vi "Update DMA Values - 321.vi"(8 "error in (no error)":errorcluster, 11 "Register Value":variant) -> (0 "error out":errorcluster, 3 "Updated DMA Values":T1[](array[typedef]) {"Data Type" format="%.0x"})   [LabVIEW 2018, in "FPGA Addon Shared.lvlib"]
uses:
  FPGA Addon Shared.lvlib
  Types/DMA Information.ctl
  Types/FPGA Addon Data Type.ctl
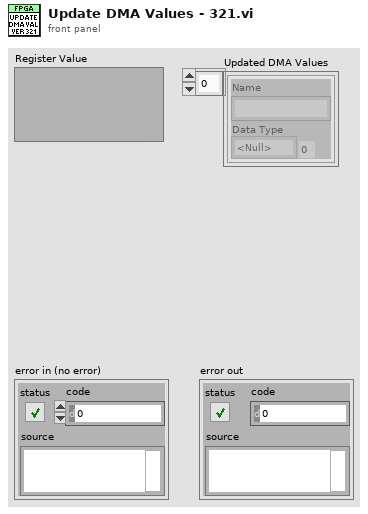
[diagram p1: front panel]
types:
  T1 = typedef "FPGA Addon Shared.lvlib/DMA Information.ctl" = cluster{"Name":string, "Data Type":T2}
  T2 = typedef "FPGA Addon Shared.lvlib/FPGA Addon Data Type.ctl" = enum8{"<Null>", "I8", "I16", "I32", "I64", "U8", "U16", "U32", "U64", "SGL", "Boolean", "Analog PWM In Settings", "Analog PWM In", "Digital PWM In Settings", "Digital PWM In", "Digital PWM Out", "Sine Out", "FXP", "FXP+/-24.5", "FXP+/-16.5", "FXP+/-32.8", "FXP+/-64.32", "FXP+/-16.7", "FXP+/-20.5", "FXP+/-27.5", "FXP+/-32.16", "FXP+16.3", "FXP+18.3", "Digital Static In", "Digital Static Out", "Digital Static In Settings", "Digital WSS Out", "Quad Encoder Settings", "Quad Encoder In", "Group"}
  T3 = cluster{"Name":string, "Data Type":enum8{"<Null>", "I8", "I16", "I32", "I64", "U8", "U16", "U32", "U64", "SGL", "Boolean", "Analog PWM In Settings", "Analog PWM In", "Digital PWM In Settings", "Digital PWM In", "Digital PWM Out", "Sine Out", "FXP+/-24.5", "FXP+/-16.5", "FXP+/-32.8", "FXP+/-64.32", "FXP+/-16.7", "FXP+/-20.5", "FXP+/-27.5", "FXP+/-32.16", "FXP+16.3", "FXP+18.3", "Digital Static In", "Digital Static Out", "Digital Static In Settings", "Digital WSS Out", "Quad Encoder Settings", "Quad Encoder In", "Group"}}[]
  T4 = enum8{"<Null>", "I8", "I16", "I32", "I64", "U8", "U16", "U32", "U64", "SGL", "Boolean", "Analog PWM In Settings", "Analog PWM In", "Digital PWM In Settings", "Digital PWM In", "Digital PWM Out", "Sine Out", "FXP+/-24.5", "FXP+/-16.5", "FXP+/-32.8", "FXP+/-64.32", "FXP+/-16.7", "FXP+/-20.5", "FXP+/-27.5", "FXP+/-32.16", "FXP+16.3", "FXP+18.3", "Digital Static In", "Digital Static Out", "Digital Static In Settings", "Digital WSS Out", "Quad Encoder Settings", "Quad Encoder In", "Group"}
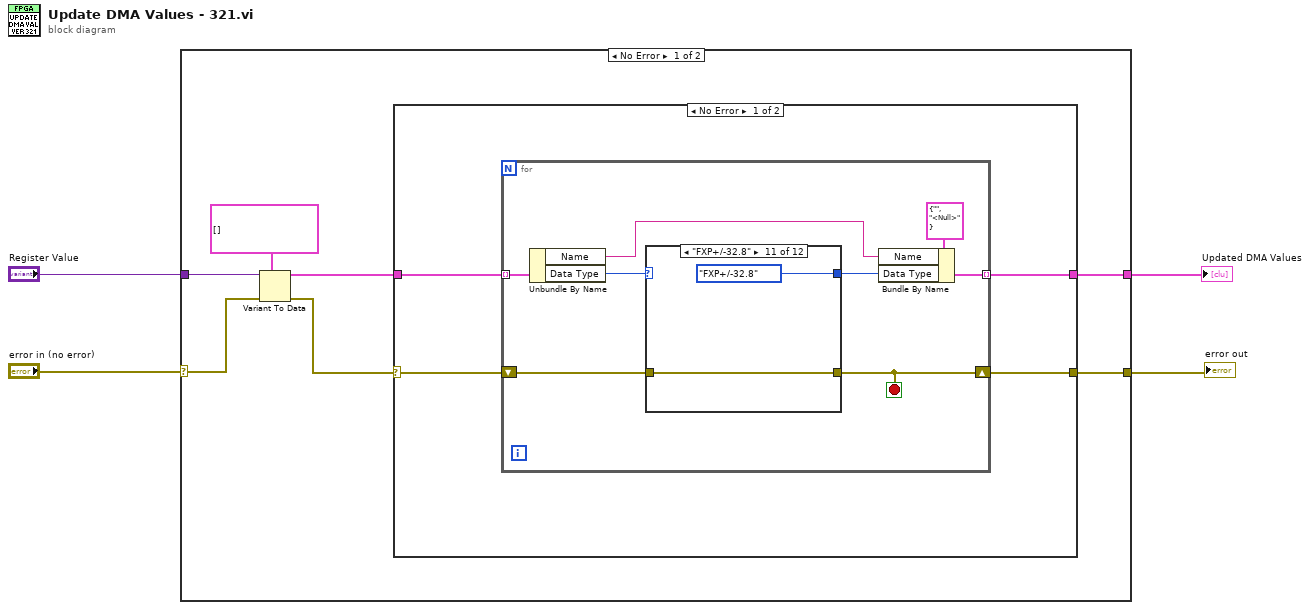
[diagram p0: block diagram]
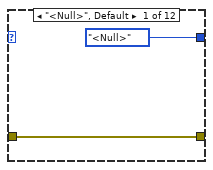
[diagram p2: hidden frame]
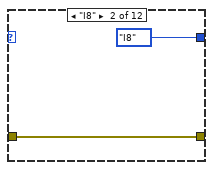
[diagram p3: hidden frame]
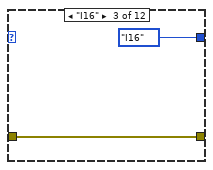
[diagram p4: hidden frame]
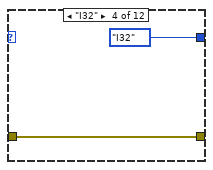
[diagram p5: hidden frame]
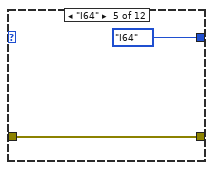
[diagram p6: hidden frame]
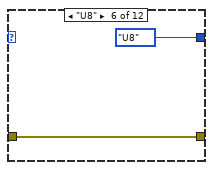
[diagram p7: hidden frame]
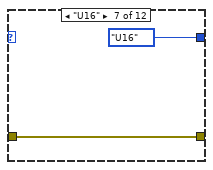
[diagram p8: hidden frame]
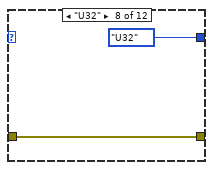
[diagram p9: hidden frame]
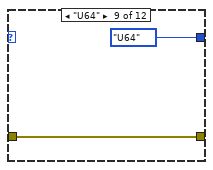
[diagram p10: hidden frame]
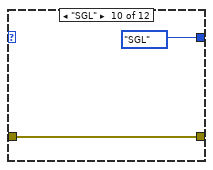
[diagram p11: hidden frame]
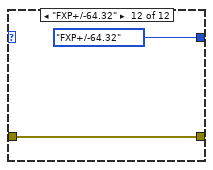
[diagram p12: hidden frame]
diagram:
  n1 = case shown="No Error" "error in (no error)" {
    selector: "error in (no error)" -> [w8 w49]
    tunnel: [w11 _] -> w1
    tunnel: "Register Value" -> [w9 _]
    tunnel: [w6 w49] -> w2
    frame No Error {
      n2 = Variant To Data(error in=w8, type=T3 [] ("Available DMA"), Variant=w9) -> (data=w10:T3, error out=w7:errorcluster)
      n3 = case shown="No Error" w7 {
        selector: w7 -> [w13 w48]
        tunnel: [w15 _] -> w11
        tunnel: w10 -> [w14 _]
        tunnel: [w12 w48] -> w6
        frame No Error {
          n4 = for {
            tunnel: w14 -> [w23] mode=indexing
            tunnel: [w22] -> w15 mode=indexing
            shift-right: [w18] -> w12
            shift-left: w13 -> [w19]
            stop <- w18 stop-if-true
            n5 = Unbundle By Name(w23) -> ("Name"=w17:string, "Data Type"=w21:T4)
            n6 = case shown="\"FXP+/-32.8\"" w21 {
              tunnel: [FPGA_Addon_Data_Type."<Null>" ("Data Type") FPGA_Addon_Data_Type."I8" ("Data Type") FPGA_Addon_Data_Type."I16" ("Data Type") FPGA_Addon_Data_Type."I32" ("Data Type") FPGA_Addon_Data_Type."I64" ("Data Type") FPGA_Addon_Data_Type."U8" ("Data Type") FPGA_Addon_Data_Type."U16" ("Data Type") FPGA_Addon_Data_Type."U32" ("Data Type") FPGA_Addon_Data_Type."U64" ("Data Type") FPGA_Addon_Data_Type."SGL" ("Data Type") FPGA_Addon_Data_Type."FXP+/-32.8" ("Data Type") FPGA_Addon_Data_Type."FXP+/-64.32" ("Data Type")] -> w20
              tunnel: w19 -> [w24 w26 w28 w30 w32 w34 w36 w38 w40 w42 w44 w46]
              tunnel: [w24 w26 w28 w30 w32 w34 w36 w38 w40 w42 w44 w46] -> w18
              frame "<Null>", Default {
              }
              frame "I8" {
              }
              frame "I16" {
              }
              frame "I32" {
              }
              frame "I64" {
              }
              frame "U8" {
              }
              frame "U16" {
              }
              frame "U32" {
              }
              frame "U64" {
              }
              frame "SGL" {
              }
              frame "FXP+/-32.8" {
              }
              frame "FXP+/-64.32" {
              }
            }
            n7 = Bundle By Name(cluster=T1 {"Name"="", "Data Type"=enum."<Null>"} ("Cluster"), "Name"=w17, "Data Type"=w20) -> (w22:T1)
          }
        }
        frame Error {
        }
      }
    }
    frame Error {
    }
  }
  "error out" <- w2
  "Updated DMA Values" <- w1
